vi "Scan.vi"(0 "VISA resource name":refnum<visa-resource-name>, 5 "Scan Channel (1)":i32=1 min=1 max=16 step=1, 7 "Autoscan (F: Off)":bool, 11 "error in (no error)":errorcluster) -> (4 "VISA resource name out":refnum<visa-resource-name>, 15 "error out":errorcluster)   [LabVIEW 2020, in "Lake Shore Cryotronics 370.lvlib"]
doc: "This VI selects which channel to switch the scanner to and configures the autoscan feature. Functions only when the Model 3716 Scanner is installed."
uses:
  Lake Shore Cryotronics 370.lvlib
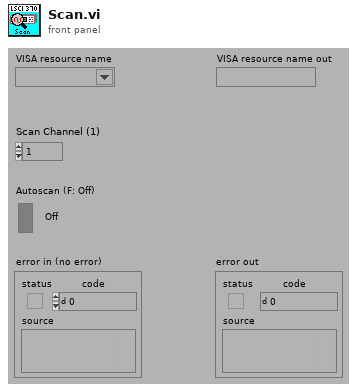
[diagram p1: front panel]
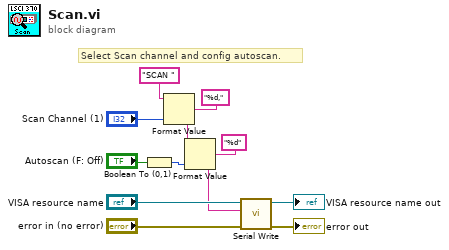
[diagram p0: block diagram]
diagram:
  # "Select Scan channel and config autoscan."
  n1 = Boolean To (0,1)(Boolean="Autoscan (F: Off)") -> (0, 1=w2:i16)
  n2 = Format Value(string ("")="SCAN ", format string="%d,", value (0)="Scan Channel (1)") -> (output string=w4:string)
  n3 = Format Value(string ("")=w4, format string="%d", value (0)=w2) -> (output string=w1:string)
  n4 = call "Serial Write.vi"("error in (no error)"="error in (no error)", "Write Buffer (\"\")"=w1, "VISA resource name"="VISA resource name") -> ("error out"=→"error out":errorcluster, "VISA resource name out"=→"VISA resource name out":refnum<visa-resource-name>)  [unwired: 6 in, 1 out]
